vi "Convert Thermocouple Reading (array).vi"(3 "Temperature Units (C)":u16(ring) items=["Celsius", "Fahrenheit", "Kelvin", "Rankine"], 5 "Thermocouple Voltage":dbl[](array[numeric]), 6 "ThermocoupleType":u16(ring)=2 items=["B", "E", "J", "K", "R", "S", "T", "N", "IC (C)", "IC (F)", "Therm."], 7 "Temperature":dbl format="%0.6f") -> (1 "Linearized Temperature":dbl[](array[numeric]))   [LabVIEW 2010]
doc: "Converts a voltage read from a thermocouple into a temperature value."
panel:
  # "National Instruments has chosen thermocouple polynomial expressions that are valid only for  particular temperature ranges (given in the VI diagram).  These polynomials come from the NIST Monograph 175.\n\nIf you wish to use a different conversion formula, you can edit this VI and enter your own equation into the appropriate formula node."
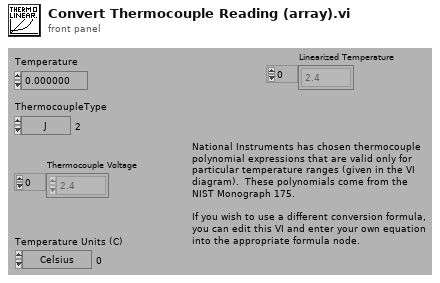
[diagram p1: front panel]
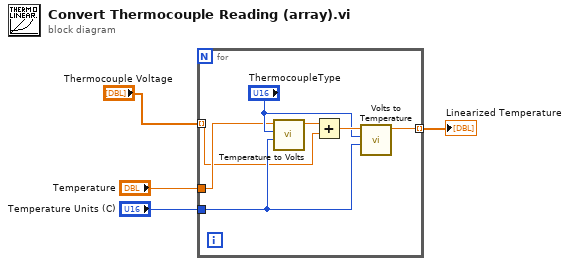
[diagram p0: block diagram]
diagram:
  n1 = for {
    tunnel: "Temperature" -> [w6]
    tunnel: [w8] -> w1 mode=indexing
    tunnel: "Thermocouple Voltage" -> [w5] mode=indexing
    tunnel: "Temperature Units (C)" -> [w7]
    n2 = call "Temperature to Volts.vi"("Temperature Units"=w7, "ThermocoupleType"="ThermocoupleType", "Temperature"=w6) -> ("Thermocouple Voltage"=w11:sgl)  [unwired: 4 in]
    n3 = Add(x=w11, y=w5) -> (x+y=w10:dbl)
    n4 = call "Volts to Temperature.vi"("Temperature Units"=w7, "ThermocoupleType"="ThermocoupleType", "Thermocouple Voltage"=w10) -> ("Temperature"=w8:sgl)  [unwired: 4 in]
  }
  "Linearized Temperature" <- w1
